vi "Symphony Test Server.vi"() -> ()   [LabVIEW 2019]
panel:
  in  "testwrite":bool
  in  "stop":bool
  in  "error in (no error)":errorcluster
  out "error out":errorcluster
  out "data":cluster{"Message":string, "Data":variant, i32}
  out "ServerConn":refnum<k13>
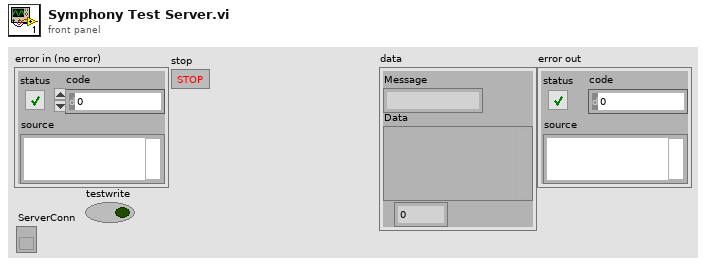
[diagram p1: front panel]
types:
  T1 = enum16{"Read", "Write", "ReadWrite", "BufferedRead", "BufferedReadWrite"}
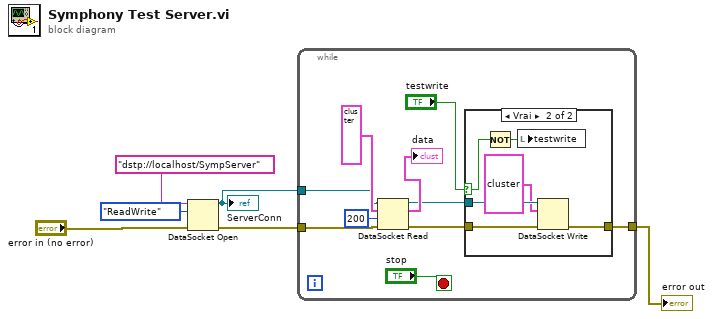
[diagram p0: block diagram]
diagram:
  n1 = DataSocket Open(8:"error in (no error)", 10:T1."ReadWrite" ("mode"), 11:"dstp://localhost/SympServer" ("URL")) -> (0:w5:errorcluster, 3:w3:refnum<k13>)  [unwired: 1 in]
  "ServerConn" <- w3
  n2 = while {
    tunnel: w5 -> [w16]
    tunnel: [w9] -> w4
    tunnel: w3 -> [w14]
    stop <- "stop" stop-if-true
    n3 = DataSocket Read(8:w16, 9:200 ("ms timeout (10000)"), 10:cluster{"Message":string, "Data":variant, i32} {"Message"="", "Data"=variant, 0} ("ClassQueue"), 11:w14) -> (0:w8:errorcluster, 2:→"data":cluster{"Message":string, "Data":variant, i32}, 3:w7:refnum<k13>)  [unwired: 1 in, 4 out]
    n4 = case shown="Vrai" "testwrite" {
      selector: "testwrite" -> [_ w19]
      tunnel: [w17 w22] -> w9
      tunnel: w8 -> [w17 w23]
      tunnel: w7 -> [_ w21]
      frame False {
      }
      frame True {
        n5 = Not(x=w19) -> (.not. x?=w18:bool)
        n6 = local write "testwrite"(w18) -> ()
        n7 = DataSocket Write(8:w23, 10:cluster{"Message":string, "Data":variant, i32} {"Message"="test1", "Data"=variant, 0} ("ClassQueue"), 11:w21) -> (0:w22:errorcluster)  [unwired: 1 in, 2 out]
      }
    }
  }
  "error out" <- w4
